vi "Library Class Children Data.vi"(7 "Destination":path, 8 "Error In":errorcluster, 11 "Library In":refnum<vi>) -> (0 "Error Out":errorcluster, 2 "Data":refnum<class "Map.lvclass">[](array[class]), 3 "Library Out":refnum<vi>)   [LabVIEW 2018, in "Scripts.lvlib"]
uses:
  Scripts.lvlib
  Toolkit/Data/Map/Map.lvclass
  Toolkit/Data/Map/Support/From String.vi
  Toolkit/Data/Map/Support/From Map Array.vi
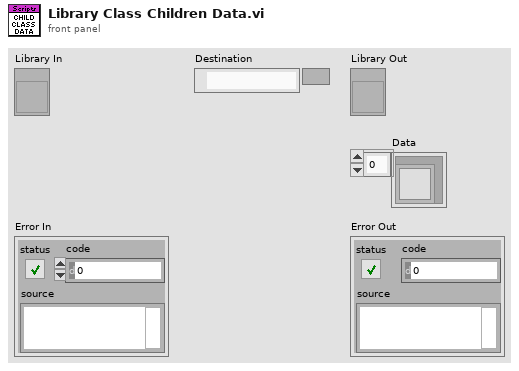
[diagram p1: front panel]
types:
  T1 = enum32{"invalid scope", "public", "private", "protected", "community"}
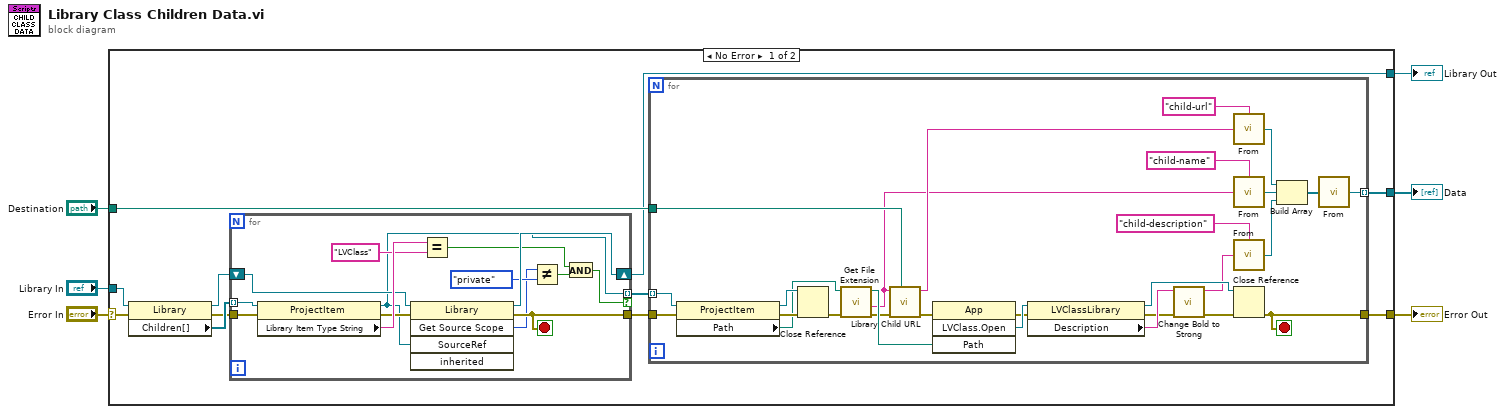
[diagram p0: block diagram]
diagram:
  n1 = case shown="No Error" "Error In" {
    selector: "Error In" -> [w13 w61]
    tunnel: [w17 w61] -> w6
    tunnel: "Destination" -> [w15 _]
    tunnel: "Library In" -> [w14 w60]
    tunnel: [w7 w60] -> w3
    tunnel: [w16 _] -> w2
    frame No Error {
      n2 = property class="Library"(reference=w14, error in=w13) -> (reference out=w8:refnum<vi>, error out=w11:errorcluster, "Children[]"=w12:refnum<vi>[])
      n3 = for {
        tunnel: w12 -> [w31] mode=indexing
        tunnel: w11 -> [w30]
        tunnel: [w23] -> w9 mode=indexing if=w21
        tunnel: [w24] -> w10
        shift-right: [w26] -> w7
        shift-left: w8 -> [w27]
        stop <- w24 stop-if-true
        n4 = property class="ProjectItem"(reference=w31, error in=w30) -> (reference out=w23:refnum<vi>, error out=w25:errorcluster, "Library Item Type String"=w29:string)
        n5 = invoke class="Library" method="Get Source Scope"(reference=w27, error in=w25, "SourceRef"=w23) -> (reference out=w26:refnum<vi>, error out=w24:errorcluster, "GetSourceScope"=w19:T1)  [unwired: 2 in, 2 out]
        n6 = Equal?(x=w29, y="LVClass") -> (x = y?=w22:bool)
        n7 = Not Equal?(x=w19, y=T1."private" ("Source Scope:Get")) -> (x != y?=w18:bool)
        n8 = And(x=w22, y=w18) -> (x .and. y?=w21:bool)
      }
      n9 = for {
        tunnel: w10 -> [w53]
        tunnel: [w54] -> w16 mode=indexing
        tunnel: [w42] -> w17
        tunnel: w15 -> [w38]
        tunnel: w9 -> [w32] mode=indexing
        stop <- w42 stop-if-true
        n10 = property class="ProjectItem"(reference=w32, error in=w53) -> (reference out=w49:refnum<vi>, error out=w50:errorcluster, "Path"=w46:path)
        n11 = Close Reference(reference=w49, error in (no error)=w50) -> (error out=w45:errorcluster)
        n12 = call <vilib>:"Get File Extension.vi"("error in (no error)"=w45, "file"=w46) -> ("error out"=w41:errorcluster, "filename without extension"=w37:string, "dup file"=w44:path)  [unwired: 5 in, 2 out]
        n13 = call "Library Child URL.vi"("Destination"=w38, "Error In"=w41, "Name"=w37) -> ("Error Out"=w40:errorcluster, "Child URL"=w39:string)  [unwired: 7 in]
        n14 = invoke class="App" method="LVClass.Open"(error in=w40, "Path"=w44) -> (error out=w47:errorcluster, "LVClass.Open"=w48:refnum<vi>)  [unwired: 2 in, 2 out]
        n15 = property class="LVClassLibrary"(reference=w48, error in=w47) -> (reference out=w43:refnum<vi>, error out=w35:errorcluster, "Description"=w36:string)
        n16 = call "Change Bold to Strong.vi"("Error In"=w35, "Bold Description"=w36) -> ("Error Out"=w34:errorcluster, "Strong Description"=w33:string)  [unwired: 8 in]
        n17 = call-poly "From.vi"("Value"=w39, "Key"="child-url") -> ("Map"=w57:refnum<class "Map.lvclass">)
        n18 = call-poly "From.vi"("Value"=w37, "Key"="child-name") -> ("Map"=w56:refnum<class "Map.lvclass">)
        n19 = call-poly "From.vi"("Value"=w33, "Key"="child-description") -> ("Map"=w51:refnum<class "Map.lvclass">)
        n20 = Close Reference(reference=w43, error in (no error)=w34) -> (error out=w42:errorcluster)
        n21 = Build Array(w57, w56, w51) -> (w55:refnum<class "Map.lvclass">[])
        n22 = call-poly "From.vi"("Maps"=w55) -> ("Map"=w54:refnum<class "Map.lvclass">)  [unwired: 1 in]
      }
    }
    frame Error {
    }
  }
  "Error Out" <- w6
  "Library Out" <- w3
  "Data" <- w2
